vi "Handshake.vi"(8 "error in (no error)":errorcluster, 11 "Connection.WS in":refnum<class "Connection.WS.lvclass">) -> (0 "error out":errorcluster, 3 "Connection.WS out":refnum<class "Connection.WS.lvclass">)   [LabVIEW 2013, in "Connection.WS_GOSPL.lvlib" / "Connection.WS.lvclass"]
uses:
  Connection.WS.lvclass
  Connection.TCP/Connection.TCP.lvclass
  Connection/Connection.lvclass/Connection.ctl
  Header Fields -- combo.ctl
  Connection.TCP/Connection.TCP.lvclass/Connection.TCP.ctl
  Connection.WS.lvclass/Connection.WS.ctl
  <vilib>/LabVIEW Open Source Project/OpenSerializer.Base64/Base64_CharSet.vi
  <vilib>/LabVIEW Open Source Project/Cryptographic Functions/SHA-1 (String).vi
  <vilib>/LabVIEW Open Source Project/Cryptographic Functions/SHA-1.vi
  <vilib>/LabVIEW Open Source Project/Cryptographic Functions/SHA-1 Pad.vi
  <vilib>/LabVIEW Open Source Project/Cryptographic Functions/SHA-1 Core.vi
  <vilib>/LabVIEW Open Source Project/Cryptographic Functions/SHA-1 Digest.vi
  <vilib>/LabVIEW Open Source Project/OpenSerializer.Base64/Serializer.Base64.lvclass
  Connection/Connection.lvclass
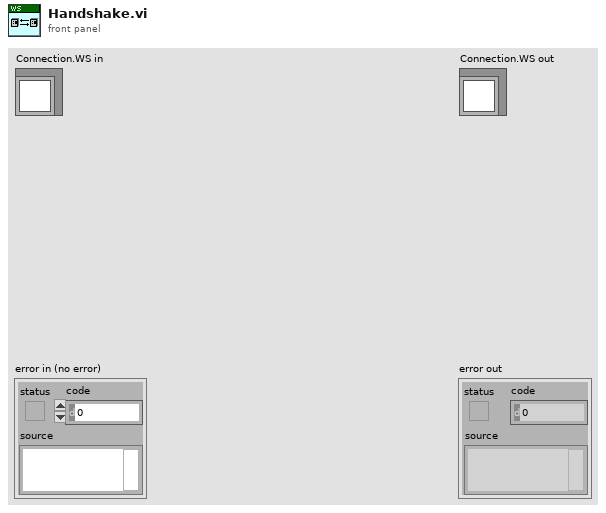
[diagram p1: front panel]
types:
  T1 = typedef "Connection.WS_GOSPL.lvlib/Connection.WS.lvclass/Header Fields -- combo.ctl" = string
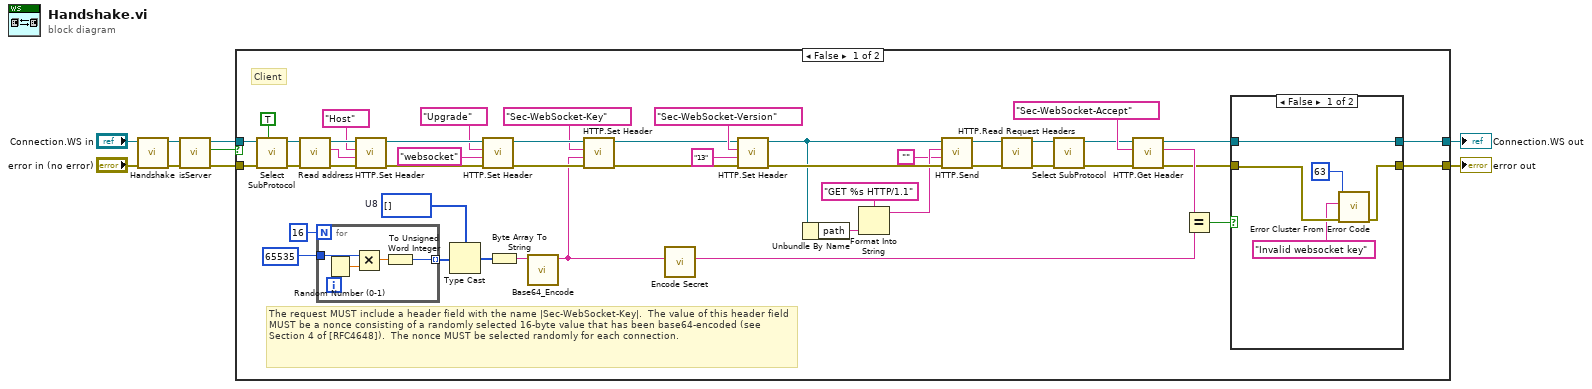
[diagram p0: block diagram]
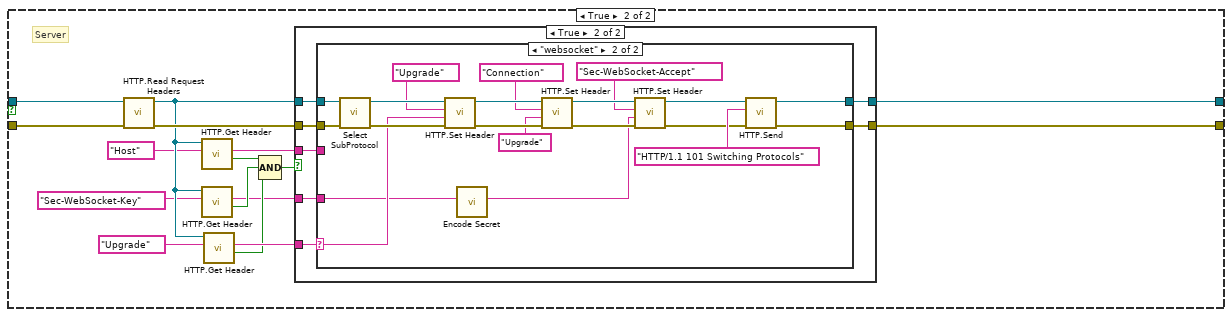
[diagram p3: hidden frame]
diagram:
  n1 = call-parent "Handshake.vi"("error in (no error)"="error in (no error)", "Connection in"="Connection.WS in") -> ("error out"=w3:errorcluster, "Connection out"=w5:refnum<class "Connection.WS.lvclass">)  [unwired: 8 in]
  n2 = call "isServer.vi"("error in (no error)"=w3, "Connection in"=w5) -> ("error out"=w2:errorcluster, "server"=w1:bool, "Connection out"=w4:refnum<class "Connection.WS.lvclass">)  [unwired: 7 in]
  n3 = case shown="False" w1 {
    tunnel: [w13 w77] -> w7
    tunnel: [w10 w76] -> w6
    tunnel: w4 -> [w37 w72]
    tunnel: w2 -> [w35 w71]
    frame False {
      w28 = u8[] []  # U8
      # "Client"
      # "The request MUST include a header field with the name |Sec-WebSocket-Key|.  The value of this header field MUST be a nonce consisting of a randomly selected 16-byte value that has been base64-encoded (see Section 4 of [RFC4648]).  The nonce MUST be selected randomly for each connection."
      n4 = call "Select SubProtocol.vi"("Set?"=TRUE, "error in (no error)"=w35, "Connection.WS in"=w37) -> ("error out"=w34:errorcluster, "Connection.WS out"=w36:refnum<class "Connection.WS.lvclass">)  [unwired: 7 in]
      n5 = call "Read address.vi"("error in (no error)"=w34, "Connection.TCP"=w36) -> ("error out"=w54:errorcluster, "address"=w56:string, "Connection.TCP"=w55:refnum<class "Connection.WS.lvclass">)  [unwired: 7 in]
      n6 = for {
        N: 16 -> [_]
        tunnel: u16 65535 -> [w67]
        tunnel: [w64] -> w29 mode=indexing
        n7 = Random Number (0-1)() -> (number: 0 to 1=w66:dbl)
        n8 = Multiply(x=w67, y=w66) -> (x*y=w65:dbl)
        n9 = To Unsigned Word Integer(number=w65) -> (unsigned 16bit integer=w64:u16)
      }
      n10 = call "HTTP.Set Header.vi"("error in (no error)"=w54, "Value"=w56, "Header Name"=T1 "Host", "Connection.WS in"=w55) -> ("error out"=w49:errorcluster, "Connection.WS out"=w52:refnum<class "Connection.WS.lvclass">)  [unwired: 6 in]
      n11 = Type Cast(type=w28, x=w29) -> (*(type *) &x=w27:u8[])
      n12 = call "HTTP.Set Header.vi"("error in (no error)"=w49, "Value"="websocket", "Header Name"=T1 "Upgrade", "Connection.WS in"=w52) -> ("error out"=w46:errorcluster, "Connection.WS out"=w48:refnum<class "Connection.WS.lvclass">)  [unwired: 6 in]
      n13 = Byte Array To String(unsigned byte array=w27) -> (string=w26:string)
      n14 = call <vilib>:"Base64_Encode.vi"("String"=w26) -> ("Encoded String"=w17:string)  [unwired: 9 in, 1 out]
      n15 = call "HTTP.Set Header.vi"("error in (no error)"=w46, "Value"=w17, "Header Name"=T1 "Sec-WebSocket-Key", "Connection.WS in"=w48) -> ("error out"=w42:errorcluster, "Connection.WS out"=w43:refnum<class "Connection.WS.lvclass">)  [unwired: 6 in]
      n16 = call "Encode Secret.vi"("Secret"=w17) -> ("Encoded Secret"=w15:string)  [unwired: 10 in]
      n17 = call "HTTP.Set Header.vi"("error in (no error)"=w42, "Value"="13", "Header Name"=T1 "Sec-WebSocket-Version", "Connection.WS in"=w43) -> ("error out"=w41:errorcluster, "Connection.WS out"=w33:refnum<class "Connection.WS.lvclass">)  [unwired: 6 in]
      n18 = Unbundle By Name(w33) -> ("path"=w38:string)
      n19 = Format Into String(format string="GET %s HTTP/1.1", w38) -> (resulting string=w39:string)  [unwired: 2 in, 1 out]
      n20 = call "HTTP.Send.vi"("error in (no error)"=w41, "body"="", "Status LIne"=w39, "Connection.WS in"=w33) -> ("error out"=w24:errorcluster, "Connection.WS out"=w25:refnum<class "Connection.WS.lvclass">)  [unwired: 6 in]
      n21 = call "HTTP.Read Request Headers.vi"("error in (no error)"=w24, "Connection.WS in"=w25) -> ("error out"=w21:errorcluster, "Connection.WS out"=w22:refnum<class "Connection.WS.lvclass">)  [unwired: 8 in]
      n22 = call "Select SubProtocol.vi"("error in (no error)"=w21, "Connection.WS in"=w22) -> ("error out"=w18:errorcluster, "Connection.WS out"=w19:refnum<class "Connection.WS.lvclass">)  [unwired: 8 in]
      n23 = call "HTTP.Get Header.vi"("error in (no error)"=w18, "Header Name"=T1 "Sec-WebSocket-Accept", "Connection.WS in"=w19) -> ("error out"=w11:errorcluster, "Value"=w16:string, "Connection.WS out"=w12:refnum<class "Connection.WS.lvclass">)  [unwired: 5 in, 1 out]
      n24 = Equal?(x=w16, y=w15) -> (x = y?=w14:bool)
      n25 = case shown="False" w14 {
        tunnel: [w61 w63] -> w13
        tunnel: w12 -> [w61 w63]
        tunnel: w11 -> [w60 w62]
        tunnel: [w59 w62] -> w10
        frame False {
          n26 = call <vilib>:"Error Cluster From Error Code.vi"("error in (no error)"=w60, "error message (\"\")"="Invalid websocket key" ("format string"), "error code (0)"=63) -> ("error out"=w59:errorcluster)  [unwired: 6 in]
        }
        frame True {
        }
      }
    }
    frame True {
      # "Server"
      n27 = call "HTTP.Read Request Headers.vi"("error in (no error)"=w71, "Connection.WS in"=w72) -> ("error out"=w80:errorcluster, "Connection.WS out"=w73:refnum<class "Connection.WS.lvclass">)  [unwired: 8 in]
      n28 = call "HTTP.Get Header.vi"("Header Name"=T1 "Host", "Connection.WS in"=w73) -> ("found"=w83:bool, "Value"=w74:string)  [unwired: 6 in, 2 out]
      n29 = call "HTTP.Get Header.vi"("Header Name"=T1 "Sec-WebSocket-Key", "Connection.WS in"=w73) -> ("found"=w82:bool, "Value"=w75:string)  [unwired: 6 in, 2 out]
      n30 = call "HTTP.Get Header.vi"("Header Name"=T1 "Upgrade", "Connection.WS in"=w73) -> ("found"=w78:bool, "Value"=w79:string)  [unwired: 6 in, 2 out]
      n31 = Compound Arithmetic op=AND(w83, w82, w78) -> (w81:bool)
      n32 = case shown="True" w81 {
        tunnel: w73 -> [w85 w91]
        tunnel: w80 -> [w84 w90]
        tunnel: w79 -> [_ w92]
        tunnel: [w85 w89] -> w77
        tunnel: [w84 w88] -> w76
        tunnel: w75 -> [_ w87]
        tunnel: w74 -> [_ w86]
        frame False {
          # "no upgrade requested"
        }
        frame True {
          n33 = case shown="\"websocket\"" w92 {
            selector: w92 -> [_ w110]
            tunnel: w91 -> [w94 w114]
            tunnel: w90 -> [w93 w113]
            tunnel: [w94 w98] -> w89
            tunnel: [w93 w97] -> w88
            tunnel: w87 -> [_ w96]
            tunnel: w86 -> [_ _]
            frame Default {
              # "upgrade protocol not supported"
            }
            frame "websocket" {
              n34 = call "Select SubProtocol.vi"("error in (no error)"=w113, "Connection.WS in"=w114) -> ("error out"=w112:errorcluster, "Connection.WS out"=w111:refnum<class "Connection.WS.lvclass">)  [unwired: 8 in]
              n35 = call "HTTP.Set Header.vi"("error in (no error)"=w112, "Value"=w110, "Header Name"=T1 "Upgrade", "Connection.WS in"=w111) -> ("error out"=w108:errorcluster, "Connection.WS out"=w109:refnum<class "Connection.WS.lvclass">)  [unwired: 6 in]
              n36 = call "Encode Secret.vi"("Secret"=w96) -> ("Encoded Secret"=w95:string)  [unwired: 10 in]
              n37 = call "HTTP.Set Header.vi"("error in (no error)"=w108, "Value"="Upgrade", "Header Name"=T1 "Connection", "Connection.WS in"=w109) -> ("error out"=w105:errorcluster, "Connection.WS out"=w106:refnum<class "Connection.WS.lvclass">)  [unwired: 6 in]
              n38 = call "HTTP.Set Header.vi"("error in (no error)"=w105, "Value"=w95, "Header Name"=T1 "Sec-WebSocket-Accept", "Connection.WS in"=w106) -> ("error out"=w99:errorcluster, "Connection.WS out"=w101:refnum<class "Connection.WS.lvclass">)  [unwired: 6 in]
              n39 = call "HTTP.Send.vi"("error in (no error)"=w99, "Status LIne"="HTTP/1.1 101 Switching Protocols" ("format string"), "Connection.WS in"=w101) -> ("error out"=w97:errorcluster, "Connection.WS out"=w98:refnum<class "Connection.WS.lvclass">)  [unwired: 7 in]
            }
          }
        }
      }
    }
  }
  "error out" <- w6
  "Connection.WS out" <- w7
